vi "ScriptWireTerminalsConpane.vi"(7 "indicator (F)/control (T)":bool, 8 "error in (no error)":errorcluster, 9 "Enum position":T1, 10 "Value position":T1, 11 "VI in":refnum<vi>) -> (0 "error out":errorcluster, 3 "VI out":refnum<vi>)   [LabVIEW 2014]
uses:
  <vilib>/Utility/miscctls.llb/LVPositionTypeDef.ctl
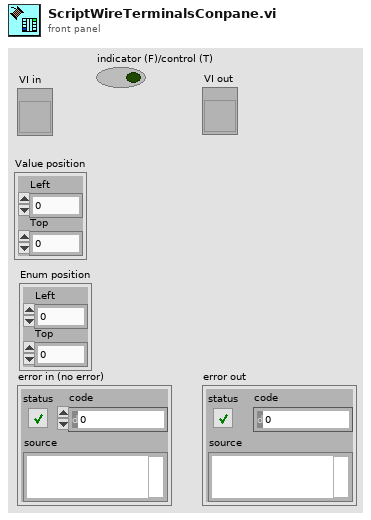
[diagram p1: front panel]
types:
  T1 = typedef "LVPositionTypeDef.ctl" = cluster{"Left":i32, "Top":i32}
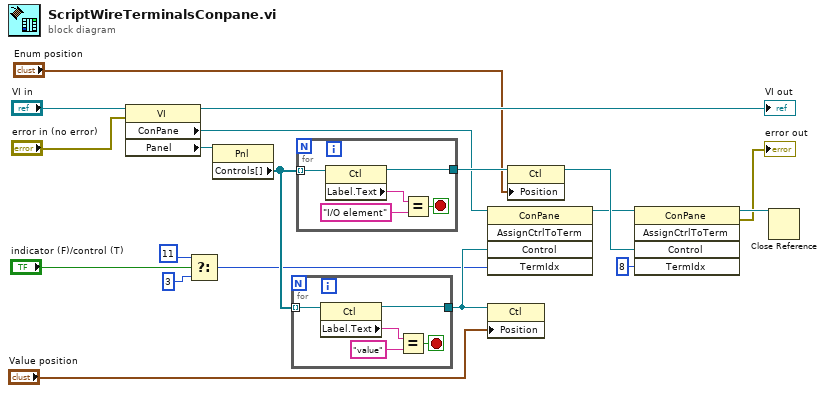
[diagram p0: block diagram]
diagram:
  n1 = property class="VI"(reference="VI in", error in="error in (no error)") -> (reference out=→"VI out":refnum<vi>, "ConPane"=w3:refnum<vi>, "Panel"=w15:refnum<vi>)  [unwired: 1 out]
  n2 = Select(t=u32 11 ("Terminal Index"), s="indicator (F)/control (T)", f=u32 3 ("Terminal Index")) -> (s? t:f=w6:u32)
  n3 = property class="Pnl"(reference=w15) -> ("Controls[]"=w16:refnum<vi>[])  [unwired: 1 in, 2 out]
  n4 = for {
    tunnel: w16 -> [w24] mode=indexing
    tunnel: [w21] -> w19
    stop <- w20 stop-if-true
    n5 = property class="Ctl"(reference=w24) -> (reference out=w21:refnum<vi>, "Label.Text"=w22:string)  [unwired: 1 in, 1 out]
    n6 = Equal?(x=w22, y="value" ("Label.Text")) -> (x = y?=w20:bool)
  }
  n7 = for {
    tunnel: w16 -> [w29] mode=indexing
    tunnel: [w26] -> w17
    stop <- w25 stop-if-true
    n8 = property class="Ctl"(reference=w29) -> (reference out=w26:refnum<vi>, "Label.Text"=w27:string)  [unwired: 1 in, 1 out]
    n9 = Equal?(x=w27, y="I/O element" ("Label.Text")) -> (x = y?=w25:bool)
  }
  n10 = invoke class="ConPane" method="AssignCtrlToTerm"(reference=w3, "Control"=w19, "TermIdx"=w6) -> (reference out=w10:refnum<vi>)  [unwired: 2 in, 4 out]
  n11 = property class="Ctl"(reference=w19, "Position"="Value position") -> ()  [unwired: 1 in, 2 out]
  n12 = property class="Ctl"(reference=w17, "Position"="Enum position") -> (reference out=w18:refnum<vi>)  [unwired: 1 in, 1 out]
  n13 = invoke class="ConPane" method="AssignCtrlToTerm"(reference=w10, "Control"=w18, "TermIdx"=u32 8 ("Terminal Index")) -> (reference out=w14:refnum<vi>, error out=→"error out":errorcluster)  [unwired: 2 in, 3 out]
  n14 = Close Reference(reference=w14) -> ()  [unwired: 1 in, 1 out]
